vi "UICtrls_BuildMessage_Array.vi"(1 "Control Label":string[](array[string]), 2 "Control Data":variant[](array[variant]), 4 "Action":T1 caption="Action (write)") -> (6 "Message":string[](array[string]), 7 "Data":variant[](array[variant]))   [LabVIEW 2025]
doc: "Build Message for UI Handler Loop for all input Controls"
uses:
  UI_Manager.lvlib
  UI_Enum_Action.ctl
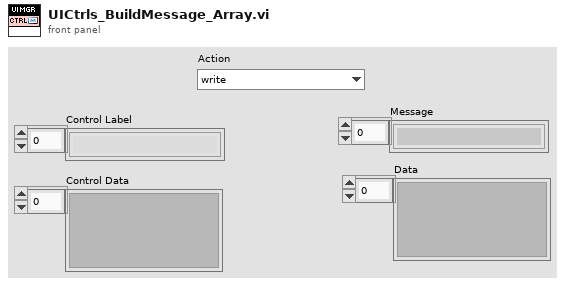
[diagram p1: front panel]
types:
  T1 = typedef "UI_Enum_Action.ctl" = enum16{"write", "disable", "visible", "read", "Numeric Set Max", "Numeric Set Min", "NamedNum Set Strings", "NamedNum Disabled Items", "WavefGraph Plot.Name", "WavefChart Plot.Name"}
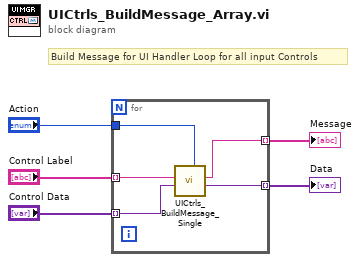
[diagram p0: block diagram]
diagram:
  # "Build Message for UI Handler Loop for all input Controls"
  n1 = for {
    tunnel: [w7] -> w5 mode=indexing
    tunnel: "Action" -> [w10]
    tunnel: "Control Data" -> [w8] mode=indexing
    tunnel: [w6] -> w2 mode=indexing
    tunnel: "Control Label" -> [w9] mode=indexing
    n2 = call "UICtrls_BuildMessage_Single.vi"("Control Label"=w9, "Control Data"=w8, "Action"=w10) -> ("Message"=w7:string, "Data"=w6:variant)  [unwired: 4 in]
  }
  "Message" <- w5
  "Data" <- w2
